vi "Run.vi"(6 "timeout":i32=2000, 7 "Name":string, 8 "error in (no error)":errorcluster, 10 "Interactive":bool, 11 "Test Runner in":refnum<class "Test Runner.lvclass">) -> (0 "error out":errorcluster, 2 "Test Suite Results":refnum<class "Test Result.lvclass">, 3 "Test Runner out":refnum<class "Test Runner.lvclass">)   [LabVIEW 2013, in "Caraya.lvlib" / "Test Runner.lvclass"]
uses:
  Test Runner.lvclass
  Test Result/Test Result.lvclass
  Test Runner.lvclass/Test Runner.ctl
  Test Suite/Define Test Suite (Default).vi
  Test Suite/Test Suite.lvclass
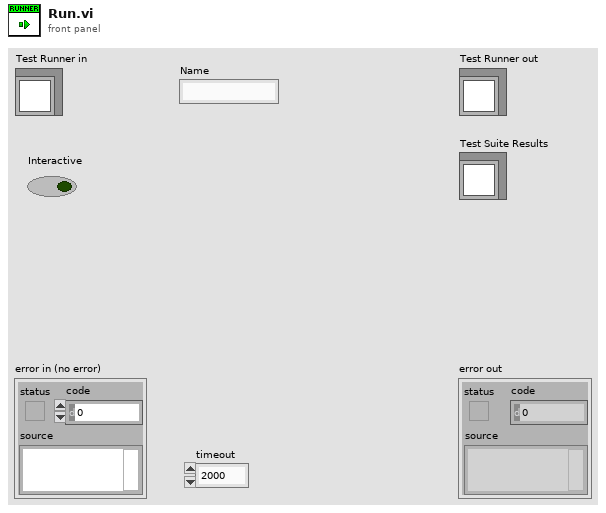
[diagram p1: front panel]
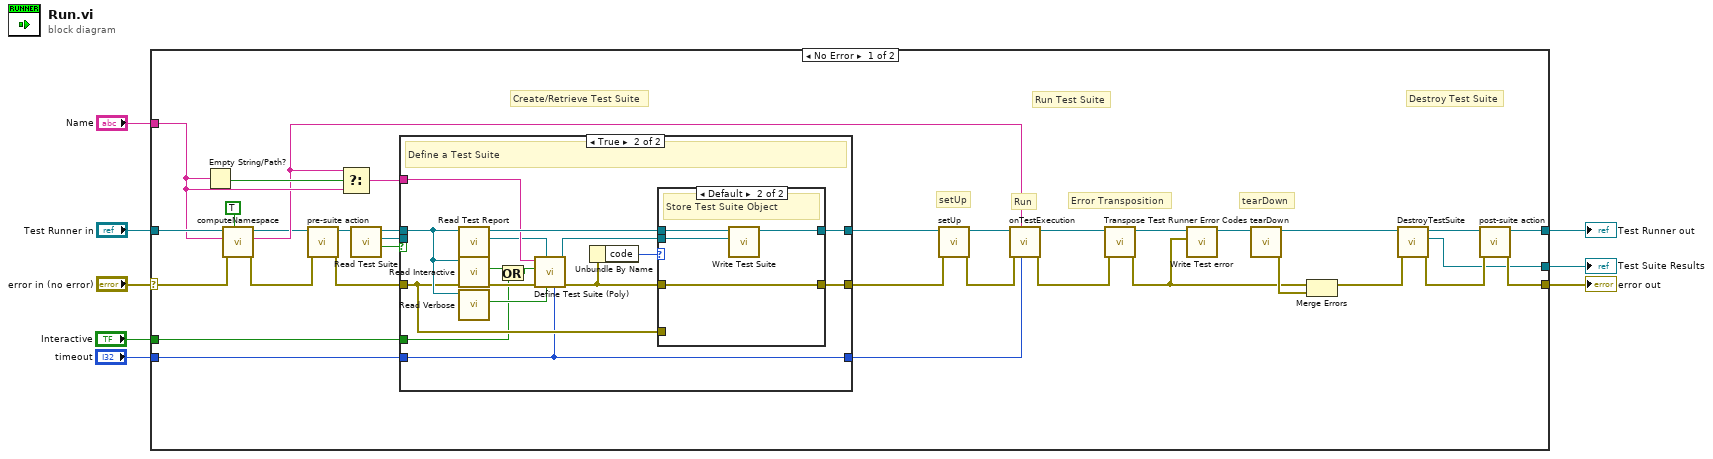
[diagram p0: block diagram]
diagram:
  n1 = case shown="No Error" "error in (no error)" {
    selector: "error in (no error)" -> [w25 w68]
    tunnel: [w12 w68] -> w7
    tunnel: [w14 w67] -> w5
    tunnel: "Test Runner in" -> [w26 w67]
    tunnel: "Interactive" -> [w27 _]
    tunnel: "Name" -> [w22 _]
    tunnel: "timeout" -> [w11 _]
    tunnel: [w9 _] -> w1
    frame No Error {
      # "Run Test Suite"
      # "Destroy Test Suite"
      # "Create/Retrieve Test Suite"
      # "Error Transposition"
      # "Run"
      # "tearDown"
      # "setUp"
      n2 = Empty String/Path?(string/path=w22) -> (empty?=w23:bool)
      n3 = call "computeNamespace.vi"("Build Namespace (F)"=TRUE, "error in (no error)"=w25, "Name"=w22, "Test Runner in"=w26) -> ("error out"=w17:errorcluster, "Namespace"=w21:string, "Test Runner out"=w19:refnum<class "Test Runner.lvclass">)  [unwired: 5 in]
      n4 = call-dynamic "pre-suite action.vi"("error in (no error)"=w17, "Test Runner in"=w19) -> ("error out"=w16:errorcluster, "Test Runner out"=w18:refnum<class "Test Runner.lvclass">)  [unwired: 8 in]
      n5 = Select(t=w21, s=w23, f=w22) -> (s? t:f=w20:string)
      n6 = call "Read Test Suite.vi"("Test Runner in"=w18) -> ("undefined"=w36:bool, "Test Suite"=w35:refnum<class "Test Suite.lvclass">, "Test Runner out"=w34:refnum<class "Test Runner.lvclass">)  [unwired: 8 in]
      n7 = case shown="True" w36 {
        tunnel: [w44 w51] -> w30
        tunnel: w34 -> [w45 w55]
        tunnel: [w45 w59] -> w33
        tunnel: w20 -> [_ w58]
        tunnel: w35 -> [_ _]
        tunnel: w16 -> [w44 w50]
        tunnel: w27 -> [_ w48]
        tunnel: w11 -> [w43 w46]
        tunnel: [w43 w46] -> w10
        frame False {
          # "Test Suite already defined"
        }
        frame True {
          # "Define a Test Suite"
          n8 = call "Read Test Report.vi"("Test Runner in"=w55) -> ("Test Report"=w56:refnum<class "Test Report.lvclass">, "Test Runner out"=w60:refnum<class "Test Runner.lvclass">)  [unwired: 8 in, 1 out]
          n9 = call "Read Interactive.vi"("Test Runner in"=w55) -> ("Interactive"=w49:bool)  [unwired: 9 in, 1 out]
          n10 = call "Read Verbose.vi"("Test Runner in"=w55) -> ("Verbose"=w54:bool)  [unwired: 9 in, 1 out]
          n11 = Or(x=w49, y=w48) -> (x .or. y?=w47:bool)
          n12 = call-poly "Define Test Suite (Poly).vi"("timeout"=w46, "Verbose (F)"=w54, "Test Report (optional)"=w56, "error in (no error)"=w50, "Interactive"=w47, "Label (VI Title)"=w58) -> ("error out"=w52:errorcluster, "Test Suite"=w57:refnum<class "Test Suite.lvclass">)  [unwired: 4 in]
          n13 = Unbundle By Name(w52) -> ("code"=w53:i32)
          n14 = case shown="Default" w53 {
            tunnel: w60 -> [w62 w66]
            tunnel: [w62 w65] -> w59
            tunnel: w57 -> [_ w64]
            tunnel: w52 -> [_ w63]
            tunnel: [w61 w63] -> w51
            tunnel: w50 -> [w61 _]
            frame 42 {
              # "error 42\nTest Suite"
              # "Already Defined"
            }
            frame Default {
              # "Store Test Suite Object"
              n15 = call "Write Test Suite.vi"("Test Suite"=w64, "Test Runner in"=w66) -> ("Test Runner out"=w65:refnum<class "Test Runner.lvclass">)  [unwired: 9 in]
            }
          }
        }
      }
      n16 = call-dynamic "setUp.vi"("error in (no error)"=w30, "Test Runner in"=w33) -> ("error out"=w28:errorcluster, "Test Runner out"=w29:refnum<class "Test Runner.lvclass">)  [unwired: 8 in]
      n17 = call-dynamic "onTestExecution.vi"("timeout (2000 ms)"=w10, "Name"=w21, "error in (no error)"=w28, "Test Runner in"=w29) -> ("error out"=w41:errorcluster, "Test Runner out"=w40:refnum<class "Test Runner.lvclass">)  [unwired: 6 in]
      n18 = call-dynamic "Transpose Test Runner Error Codes.vi"("error in (no error)"=w41, "Test Runner in"=w40) -> ("error out"=w37:errorcluster, "Test Runner out"=w42:refnum<class "Test Runner.lvclass">)  [unwired: 8 in]
      n19 = call "Write Test error.vi"("Test error"=w37, "Test Runner in"=w42) -> ("Test Runner out"=w39:refnum<class "Test Runner.lvclass">)  [unwired: 9 in]
      n20 = call-dynamic "tearDown.vi"("Test Runner in"=w39) -> ("error out"=w38:errorcluster, "Test Runner out"=w32:refnum<class "Test Runner.lvclass">)  [unwired: 9 in]
      n21 = Merge Errors(w37, w38) -> (w31:errorcluster)
      n22 = call "DestroyTestSuite.vi"("error in (no error)"=w31, "Test Runner in"=w32) -> ("error out"=w13:errorcluster, "Test Suite Results"=w9:refnum<class "Test Result.lvclass">, "Test Runner out"=w15:refnum<class "Test Runner.lvclass">)  [unwired: 7 in]
      n23 = call-dynamic "post-suite action.vi"("error in (no error)"=w13, "Test Runner in"=w15) -> ("error out"=w12:errorcluster, "Test Runner out"=w14:refnum<class "Test Runner.lvclass">)  [unwired: 8 in]
    }
    frame Error {
    }
  }
  "error out" <- w7
  "Test Runner out" <- w5
  "Test Suite Results" <- w1
